vi "Main.vi"() -> ()   [LabVIEW 2020]
uses:
  <vilib>/Utility/cursorutil.llb/Set Cursor (Icon Pict).vi
  <vilib>/Waveform/WDTOps.llb/WDT Get Waveform Time Array DBL.vi
  <vilib>/measure/NI_MABase.lvlib
panel:
  out "Limit":cluster{"Lower Limit":dbl, "Upper Limit":dbl}
  out "Overview":cluster{"X":dbl[], "Y":dbl[]}[](graph)
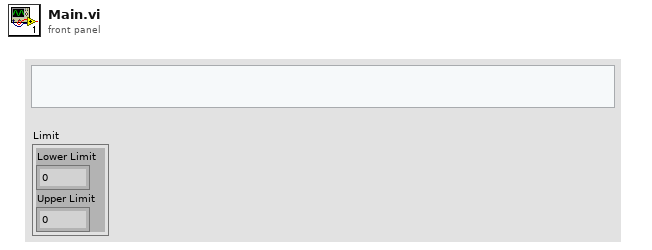
[diagram p1: front panel]
types:
  T1 = cluster{"In Span?":bool, "Span":dbl, "Drag Offset":dbl}
  T2 = typedef "LVPoint32TypeDef.ctl" = cluster{"Horizontal":i32, "Vertical":i32}
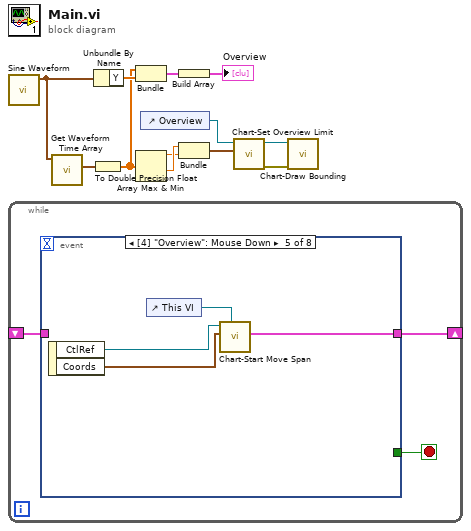
[diagram p0: block diagram]
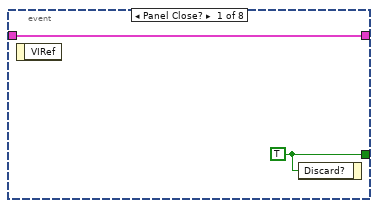
[diagram p2: hidden frame]
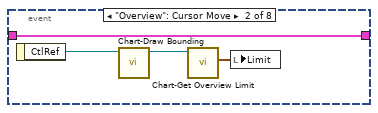
[diagram p3: hidden frame]
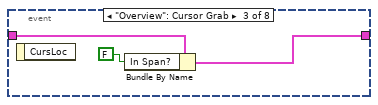
[diagram p4: hidden frame]
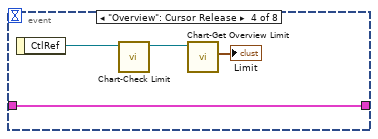
[diagram p5: hidden frame]
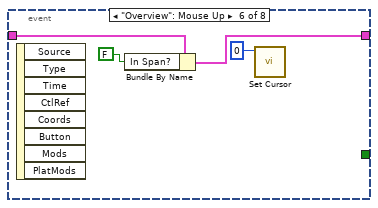
[diagram p6: hidden frame]
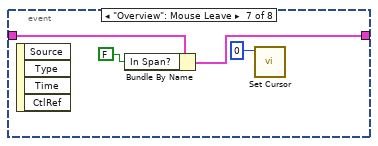
[diagram p7: hidden frame]
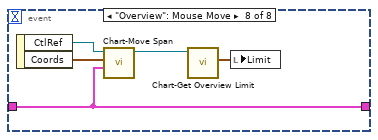
[diagram p8: hidden frame]
diagram:
  n1 = call <vilib>:"Sine Waveform.vi"() -> ("signal out"=w12:waveform(dbl))  [unwired: 10 in, 1 out]
  n2 = while {
    shift-right: [w14] -> _
    shift-left: _ -> [w13]
    stop <- w15 stop-if-true
    n3 = event shown="[4] \"Overview\": Mouse Down" {
      selector: _ -> [_ _ _ _ _ _ _ _]
      dyn-events: _ -> [_ _ _ _ _ _ _ _]
      timeout: _ -> [_ _ _ _ _ _ _ _]
      tunnel: [w17 _ _ _ _ _ _ _] -> w15
      tunnel: [w16 w18 w22 w25 w29 w33 w37 w44] -> w14
      tunnel: w13 -> [w16 w18 w23 w25 _ w35 w39 w44]
      event Panel Close? {
        w17 = TRUE ("Discard?")
        n4 = event-data() -> ()  [unwired: 1 in, 1 out]
        n5 = event-data("Discard?"=w17) -> ()  [unwired: 1 in, 1 out]
      }
      event "Overview": Cursor Move {
        n6 = event-data() -> ("CtlRef"=w21:refnum<vi>)  [unwired: 1 in]
        n7 = call "Chart-Draw Bounding.vi"("XY Graph Ref In"=w21) -> ("XY Graph Ref Out"=w20:refnum<vi>)  [unwired: 9 in, 1 out]
        n8 = call "Chart-Get Overview Limit.vi"("Overview Refnum In"=w20) -> ("Limit"=w19:cluster{"Lower Limit":dbl, "Upper Limit":dbl})  [unwired: 8 in, 2 out]
        n9 = local write "Limit"(w19) -> ()
      }
      event "Overview": Cursor Grab {
        n10 = event-data() -> ()  [unwired: 1 in, 1 out]
        n11 = Bundle By Name(cluster=w23, "In Span?"=FALSE) -> (w22:T1)
      }
      event "Overview": Cursor Release {
        n12 = event-data() -> ("CtlRef"=w27:refnum<vi>)  [unwired: 1 in]
        n13 = call "Chart-Check Limit.vi"("XY Graph Ref In"=w27) -> ("XY Graph Ref Out"=w26:refnum<vi>)  [unwired: 9 in, 1 out]
        n14 = call "Chart-Get Overview Limit.vi"("Overview Refnum In"=w26) -> ("Limit"=→"Limit":cluster{"Lower Limit":dbl, "Upper Limit":dbl})  [unwired: 8 in, 2 out]
      }
      event "Overview": Mouse Down {
        n15 = event-data() -> ("CtlRef"=w32:refnum<vi>, "Coords"=w31:T2)  [unwired: 1 in]
        n16 = control-ref of="This VI"() -> (w30:refnum<vi>)
        n17 = call "Chart-Start Move Span.vi"("VI reference (current VI)"=w30, "Coords"=w31, "XY Graph Ref In"=w32) -> ("Information"=w29:T1)  [unwired: 6 in, 2 out]
      }
      event "Overview": Mouse Up {
        n18 = event-data() -> ()  [unwired: 1 in, 8 out]
        n19 = Bundle By Name(cluster=w35, "In Span?"=FALSE) -> (w33:T1)
        n20 = call-poly <vilib>:"Set Cursor.vi"("icon"=u16 0) -> ()  [unwired: 9 in, 2 out]
      }
      event "Overview": Mouse Leave {
        n21 = event-data() -> ()  [unwired: 1 in, 4 out]
        n22 = Bundle By Name(cluster=w39, "In Span?"=FALSE) -> (w37:T1)
        n23 = call-poly <vilib>:"Set Cursor.vi"("icon"=u16 0) -> ()  [unwired: 9 in, 2 out]
      }
      event "Overview": Mouse Move {
        n24 = event-data() -> ("CtlRef"=w45:refnum<vi>, "Coords"=w43:T2)  [unwired: 1 in]
        n25 = call "Chart-Move Span.vi"("Information"=w44, "Coords"=w43, "XY Graph Ref In"=w45) -> ("XY Graph Ref Out"=w41:refnum<vi>)  [unwired: 7 in, 1 out]
        n26 = call "Chart-Get Overview Limit.vi"("Overview Refnum In"=w41) -> ("Limit"=w42:cluster{"Lower Limit":dbl, "Upper Limit":dbl})  [unwired: 8 in, 2 out]
        n27 = local write "Limit"(w42) -> ()
      }
    }
  }
  n28 = call-poly <vilib>:"Get Waveform Time Array.vi"("waveform in"=w12) -> ("X array"=w11:timestamp[])  [unwired: 9 in, 1 out]
  n29 = To Double Precision Float(number=w11) -> (double precision float=w6:dbl[])
  n30 = Unbundle By Name(w12) -> ("Y"=w10:dbl[])
  n31 = Bundle(w6, "Y"=w10) -> (w9:cluster{dbl[], "Y":dbl[]})  [unwired: 1 in]
  n32 = Array Max & Min(array=w6) -> (max value=w4:dbl, min value=w5:dbl)  [unwired: 2 out]
  n33 = control-ref of="Overview"() -> (w7:refnum<vi>)
  n34 = Build Array(w9) -> (→"Overview":cluster{dbl[], "Y":dbl[]}[])
  n35 = Bundle(w5, w4) -> (w3:cluster{dbl, dbl})  [unwired: 1 in]
  n36 = call "Chart-Set Overview Limit.vi"("Limit"=w3, "Overview Refnum In"=w7) -> ("error out"=w1:errorcluster, "Overview Refnum Out"=w2:refnum<vi>)  [unwired: 8 in]
  n37 = call "Chart-Draw Bounding.vi"("error in (no error)"=w1, "XY Graph Ref In"=w2) -> ()  [unwired: 8 in, 2 out]
